vi "svc_Build Frequency Array.vi"(11 "spectrum":T1 {"magnitude" format="%.2f"; "df [Hz]" format="%.2f"; "f0" format="%.2f"}) -> (0 "frequency array [Hz]":dbl[](array[numeric]) format="%.2f", 1 "df [Hz]":dbl format="%.2f", 2 "f0":dbl format="%.2f", 3 "magnitude":dbl[](array[numeric]) format="%.2f")   [LabVIEW 2017]
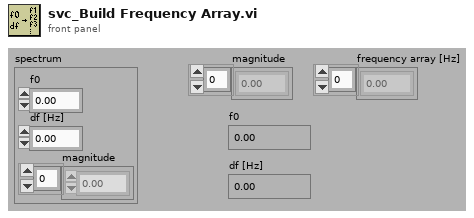
[diagram p1: front panel]
types:
  T1 = cluster{"f0":dbl, "df [Hz]":dbl, "magnitude":dbl[]}
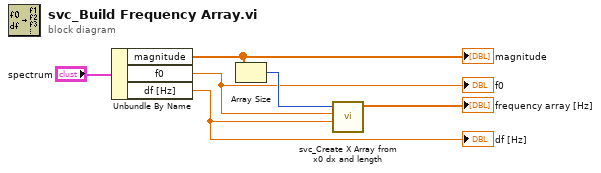
[diagram p0: block diagram]
diagram:
  n1 = Unbundle By Name("spectrum") -> ("magnitude"=w5:dbl[], "f0"=w3:dbl, "df [Hz]"=w2:dbl)
  "magnitude" <- w5
  "f0" <- w3
  "df [Hz]" <- w2
  n2 = Array Size(array=w5) -> (size(s)=w4:i32)
  n3 = call <vilib>:"svc_Create X Array from x0 dx and length.vi"("dx"=w2, "x0"=w3, "length"=w4) -> ("X"=→"frequency array [Hz]":dbl[])  [unwired: 8 in]
